vi "Memory.Pointer.Bool.New.vi"(8 "error in (no error)":errorcluster) -> (0 "error out":errorcluster, 3 "U64 Pointer":refnum<class "Memory.Pointer.Bool.lvclass">)   [LabVIEW 2016, in "LabVIEW Memory Manager.lvlib" / "Memory.Pointer.Bool.lvclass"]
uses:
  Memory.Pointer.Bool.lvclass
  C:/Users/Ryan/Documents/Git/Sourcetree/LabVIEW-Memory-Manager/Source/Library/Classes/Pointer/Memory.Pointer.lvclass
  Pointer/Memory.Pointer.lvclass/Memory.Pointer.ctl
  Pointer/Methods/Memory.Pointer.Set Address.vi
  Pointer/Methods/Memory.Pointer.Set Size.vi
  Pointer/Memory.Pointer.lvclass
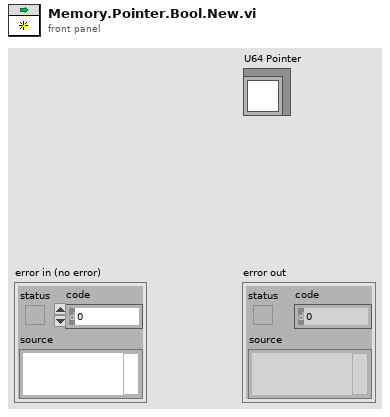
[diagram p1: front panel]
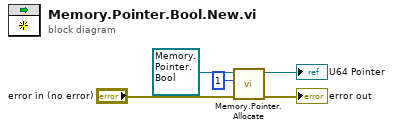
[diagram p0: block diagram]
diagram:
  n1 = call "Memory.Pointer.Allocate.vi"("error in (no error)"="error in (no error)", "size"=u64 1, "Pointer in"=refnum<class "Memory.Pointer.Bool.lvclass"> refnum ("LabVIEW Memory Manager.lvlib:DBL Pointer")) -> ("error out"=→"error out":errorcluster, "Pointer out"=→"U64 Pointer":refnum<class "Memory.Pointer.Bool.lvclass">)  [unwired: 6 in, 1 out]
